vi "sample.vi"() -> ()   [LabVIEW 2019]
panel:
  out "instrument driver revision":string caption="Instrument driver revision"
  out "Slot Configuration":string[](array[string])
  out "error out":errorcluster
  in  "resource name":refnum<visa-resource-name>="COM4"
  in  "error in (no error)":errorcluster {"code" format="%.0x"}
  out "Firmware Revision":string
  out "Instrument Name":string
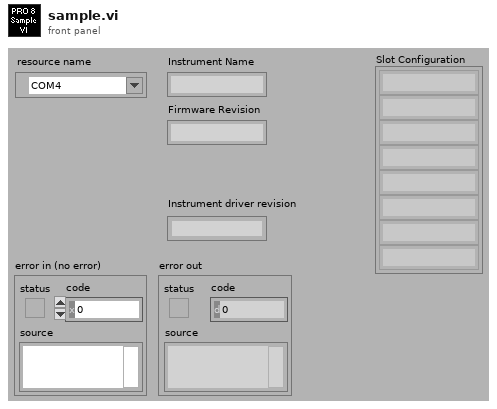
[diagram p1: front panel]
types:
  T1 = cluster{"Slot 1 Type":i16, "Slot 2 Type":i16, "Slot 3 Type":i16, "Slot 4 Type":i16, "Slot 5 Type":i16, "Slot 6 Type":i16, "Slot 7 Type":i16, "Slot 8 Type":i16}
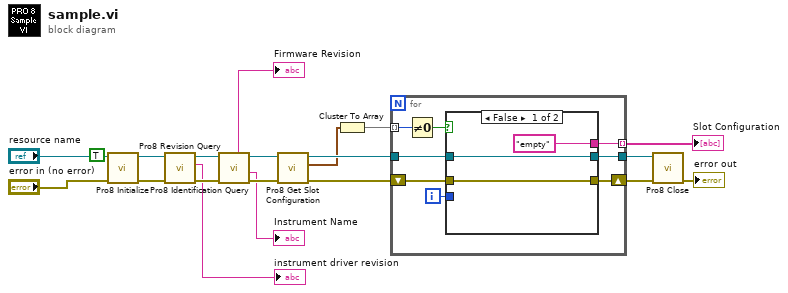
[diagram p0: block diagram]
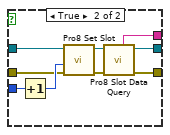
[diagram p2: hidden frame]
diagram:
  n1 = call <instrlib>:"Pro8 Initialize.vi"("error in (no error)"="error in (no error)", "id query (Do Query)"=TRUE, "resource name"="resource name") -> ("error out"=w6:errorcluster, "instrument handle out"=w8:refnum<visa-resource-name>)  [unwired: 7 in]
  n2 = call <instrlib>:"Pro8 Revision Query.vi"("error in (no error)"=w6, "instrument handle"=w8) -> ("error out"=w5:errorcluster, "instrument driver revision"=→"instrument driver revision":string, "instrument handle out"=w7:refnum<visa-resource-name>)  [unwired: 6 in, 1 out]
  n3 = call <instrlib>:"Pro8 Identification Query.vi"("error in (no error)"=w5, "instrument handle"=w7) -> ("error out"=w18:errorcluster, "Instrument Name"=→"Instrument Name":string, "instrument handle out"=w17:refnum<visa-resource-name>, "Firmware Revision"=→"Firmware Revision":string)  [unwired: 4 in, 2 out]
  n4 = call <instrlib>:"Pro8 Get Slot Configuration.vi"("error in (no error)"=w18, "instrument handle"=w17) -> ("error out"=w20:errorcluster, "Slot Type"=w3:T1, "instrument handle out"=w19:refnum<visa-resource-name>)  [unwired: 6 in, 1 out]
  n5 = Cluster To Array(cluster=w3) -> (array=w2:i16[])
  n6 = for {
    tunnel: w19 -> [w26]
    tunnel: [w23] -> w14
    shift-right: [w24] -> w13
    shift-left: w20 -> [w25]
    tunnel: [w22] -> w9 mode=indexing
    tunnel: w2 -> [w21] mode=indexing
    i -> [w27]
    n7 = Not Equal To 0?(x=w21) -> (x != 0?=w28:bool)
    n8 = case shown="False" w28 {
      tunnel: w27 -> [_ w40]
      tunnel: ["empty" w36] -> w22
      tunnel: [w30 w35] -> w24
      tunnel: [w31 w34] -> w23
      tunnel: w26 -> [w31 w33]
      tunnel: w25 -> [w30 w32]
      frame False {
      }
      frame True {
        n9 = Increment(x=w40) -> (x+1=w39:i32)
        n10 = call <instrlib>:"Pro8 Set Slot.vi"("error in (no error)"=w32, "Slot (1)"=w39, "instrument handle"=w33) -> ("error out"=w37:errorcluster, "instrument handle out"=w38:refnum<visa-resource-name>)  [unwired: 7 in]
        n11 = call <instrlib>:"Pro8 Slot Data Query.vi"("error in (no error)"=w37, "instrument handle"=w38) -> ("error out"=w35:errorcluster, "instrument handle out"=w34:refnum<visa-resource-name>, "Identification String"=w36:string)  [unwired: 4 in, 3 out]
      }
    }
  }
  "Slot Configuration" <- w9
  n12 = call <instrlib>:"Pro8 Close.vi"("error in (no error)"=w13, "instrument handle"=w14) -> ("error out"=→"error out":errorcluster)  [unwired: 9 in]
